vi "getViConnect.vi"(8 "error in (no error)":errorcluster, 11 "LibReader in":refnum<class "LibReader.lvclass">) -> (0 "error out":errorcluster, 2 "pathViConnect":path, 3 "LibReader out":refnum<class "LibReader.lvclass">)   [LabVIEW 2018, in "LibReader.lvclass"]
doc: "Get the path of connect vi."
uses:
  LibReader.lvclass
  LibReader.lvclass/LibReader.ctl
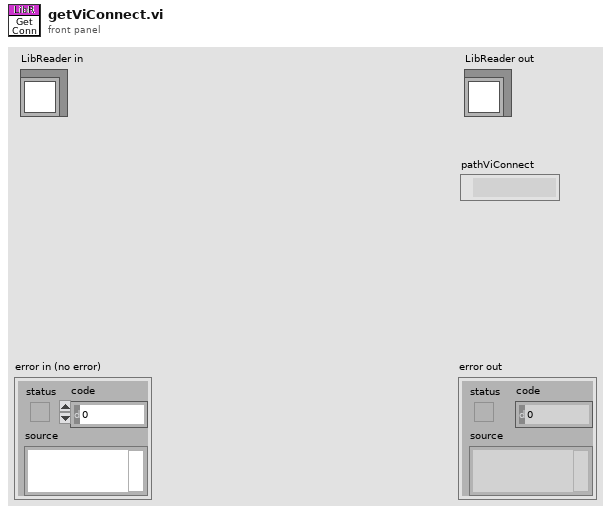
[diagram p1: front panel]
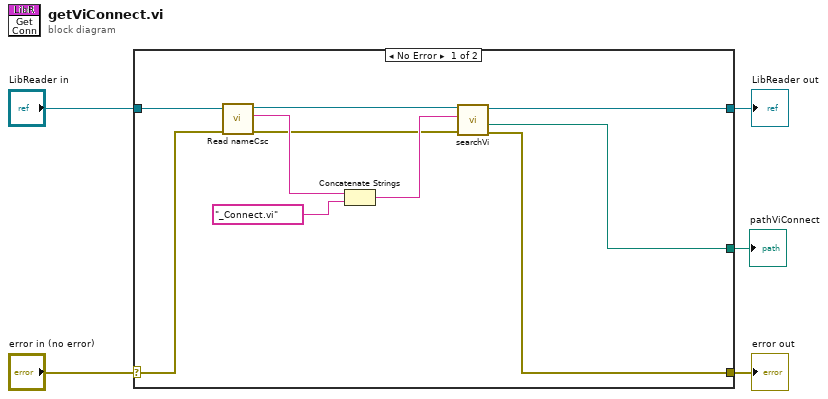
[diagram p0: block diagram]
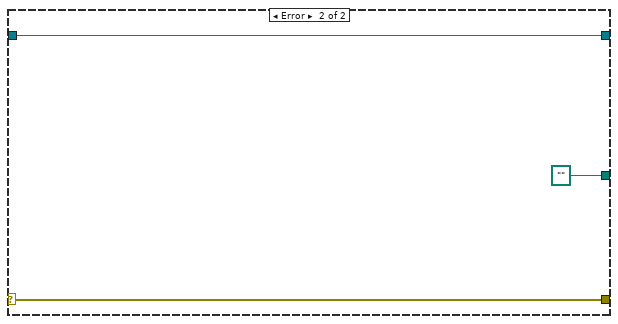
[diagram p2: hidden frame]
diagram:
  n1 = case shown="No Error" "error in (no error)" {
    selector: "error in (no error)" -> [w11 w18]
    tunnel: [w14 w18] -> w4
    tunnel: [w13 w17] -> w2
    tunnel: "LibReader in" -> [w12 w17]
    tunnel: [w15 path "" ("pathVi")] -> w1
    frame No Error {
      n2 = call "Read nameCsc.vi"("error in (no error)"=w11, "LibReader in"=w12) -> ("error out"=w6:errorcluster, "nameCsc"=w9:string, "LibReader out"=w10:refnum<class "LibReader.lvclass">)  [unwired: 7 in]
      n3 = Concatenate Strings(w9, "_Connect.vi" ("regExpr")) -> (w7:string)
      n4 = call "searchVi.vi"("error in (no error)"=w6, "regExpr"=w7, "LibReader in"=w10) -> ("error out"=w14:errorcluster, "pathVi"=w15:path, "LibReader out"=w13:refnum<class "LibReader.lvclass">)  [unwired: 5 in, 1 out]
    }
    frame Error {
    }
  }
  "error out" <- w4
  "LibReader out" <- w2
  "pathViConnect" <- w1
